vi "QCA - DUT Receive.vi"(0 "CART TCP Connection In":refnum<k5>, 1 "Rx_Test Parameters":T1 {"OFDM Data Rate (Mbps)" items=["6", "9", "12", "18", "24", "36", "48", "54"]; "DSSS Data Rate (Mbps)" items=["1", "2", "5.5 CCK", "5.5 PBCC", "11 CCK", "11 PBCC", "22", "33"]; "80211n PLCP Frame Format" items=["Mixed Format", "Greenfield Format"]}, 11 "error in (no error)":errorcluster) -> (4 "CART TCP Connection Out":refnum<k5>, 6 "Messages Logged":string[](array[string]), 14 "Command Sent":string, 15 "error out":errorcluster)   [LabVIEW 2011]
uses:
  TV/RW/Includes/WLAN - TV - RW - INC - RxTestParameters.ctl
  Controls/Data Rates.ctl
panel:
  in  "OFDM Data Rate (Mbps)":i32(ring) items=["6", "9", "12", "18", "24", "36", "48", "54"]
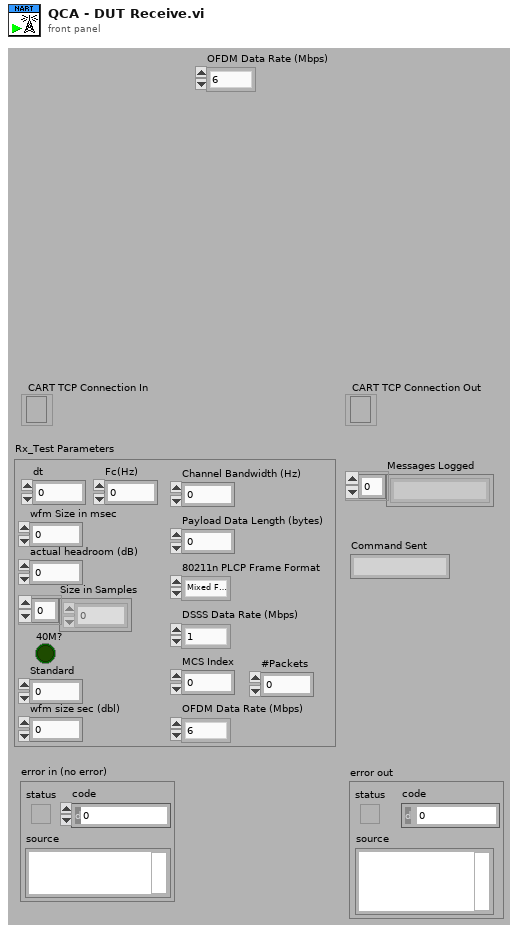
[diagram p1: front panel]
types:
  T1 = typedef "WLAN - TV - RW - INC - RxTestParameters.ctl" = cluster{"wfm Size in msec":i32, "actual headroom (dB)":dbl, "Size in Samples":i32[], "40M?":bool, "Standard ":i32, "wfm size sec (dbl)":dbl, "dt":dbl, "Channel Bandwidth (Hz)":dbl, "Payload Data Length (bytes)":i32, "80211n PLCP Frame Format":i32, "DSSS Data Rate (Mbps)":i32, "OFDM Data Rate (Mbps)":i32, "MCS Index":i32, "Fc(Hz)":dbl, "#Packets":i32}
  T2 = typedef "Data Rates.ctl" = string
  T3 = cluster{"Frequency, MHz":u32, "Data Rate":T2, "Packet Count":i32, "RX Mac Address":string, "TX Mac Address":string, "BS Mac Address":string, "Packet Length":u32, "Broadcast":bool}
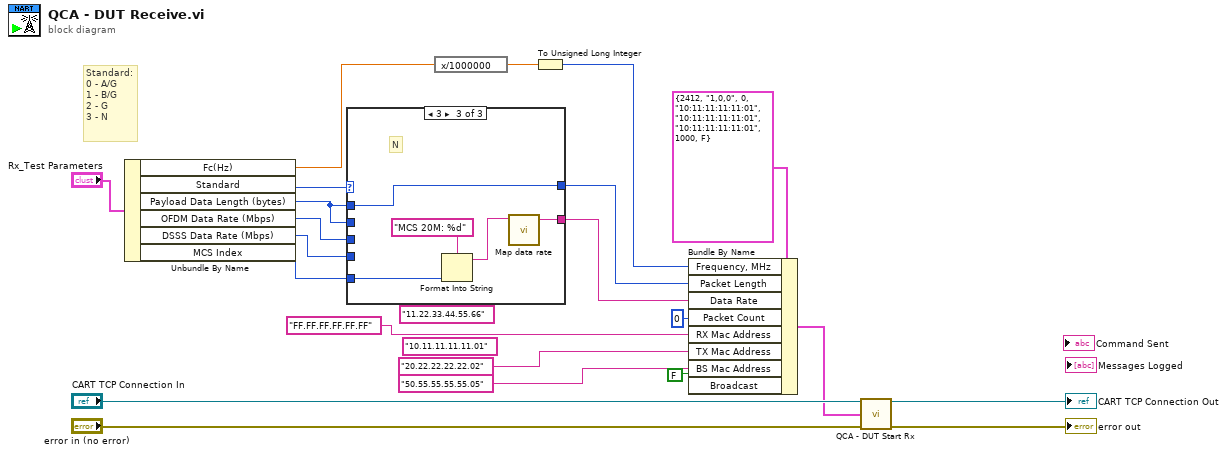
[diagram p0: block diagram]
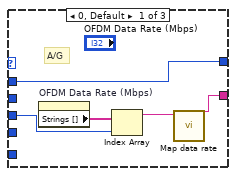
[diagram p2: hidden frame]
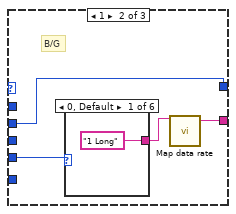
[diagram p3: hidden frame]
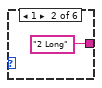
[diagram p4: hidden frame]
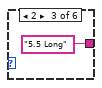
[diagram p5: hidden frame]
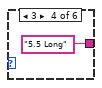
[diagram p6: hidden frame]
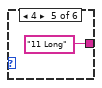
[diagram p7: hidden frame]
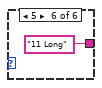
[diagram p8: hidden frame]
diagram:
  (unwired) "11.22.33.44.55.66" ("RX Mac")
  (unwired) "10.11.11.11.11.01" ("RX Mac")
  # "Standard:\n0 - A/G\n1 - B/G\n2 - G\n3 - N"
  n1 = Unbundle By Name("Rx_Test Parameters") -> ("Fc(Hz)"=w4:dbl, "Standard"=w12:i32, "Payload Data Length (bytes)"=w11:i32, "OFDM Data Rate (Mbps)"=w10:i32, "DSSS Data Rate (Mbps)"=w9:i32, "MCS Index"=w8:i32)
  n2 = case shown="3" w12 {
    tunnel: [w27 w31 w42] -> w7
    tunnel: w11 -> [w27 _ w42]
    tunnel: w11 -> [_ w31 _]
    tunnel: w10 -> [w23 _ _]
    tunnel: w9 -> [_ w30 _]
    tunnel: w8 -> [_ _ w40]
    tunnel: [w26 w29 w41] -> w6
    frame 0, Default {
      # "A/G"
      n3 = property on="OFDM Data Rate (Mbps)" class="Ring (strict)"() -> ("Strings []"=w25:string[])  [unwired: 2 in, 2 out]
      n4 = Index Array(array=w25, index=w23) -> (element=w24:string)
      n5 = call "Map data rate.vi"("Data Rate In"=w24) -> ("Data Rate Out"=w26:string)  [unwired: 10 in]
    }
    frame 1 {
      # "B/G"
      n6 = case shown="0, Default" w30 {
        tunnel: ["1 Long" ("Data Rate In") "2 Long" ("Data Rate In") "5.5 Long" ("Data Rate In") "5.5 Long" ("Data Rate In") "11 Long" ("Data Rate In") "11 Long" ("Data Rate In")] -> w28
        frame 0, Default {
        }
        frame 1 {
        }
        frame 2 {
        }
        frame 3 {
        }
        frame 4 {
        }
        frame 5 {
        }
      }
      n7 = call "Map data rate.vi"("Data Rate In"=w28) -> ("Data Rate Out"=w29:string)  [unwired: 10 in]
    }
    frame 3 {
      # "N"
      n8 = Format Into String(format string="MCS 20M: %d", w40) -> (resulting string=w38:string)  [unwired: 2 in, 1 out]
      n9 = call "Map data rate.vi"("Data Rate In"=w38) -> ("Data Rate Out"=w41:string)  [unwired: 10 in]
    }
  }
  n10 = expression code="x/1000000"(w4) -> (w17:dbl)
  n11 = To Unsigned Long Integer(number=w17) -> (unsigned 32bit integer=w16:u32)
  n12 = Bundle By Name(cluster=T3 {"Frequency, MHz"=2412, "Data Rate"="1,0,0", "Packet Count"=0, "RX Mac Address"="10:11:11:11:11:01", "TX Mac Address"="10:11:11:11:11:01", "BS Mac Address"="10:11:11:11:11:01", "Packet Length"=1000, "Broadcast"=FALSE} ("Receive Config"), "Frequency, MHz"=w16, "Packet Length"=w7, "Data Rate"=w6, "Packet Count"=0, "RX Mac Address"="FF.FF.FF.FF.FF.FF" ("RX Mac"), "TX Mac Address"="20.22.22.22.22.02" ("RX Mac"), "BS Mac Address"="50.55.55.55.55.05" ("RX Mac"), "Broadcast"=FALSE ("ART2 Data.Receive Config.Broadcast")) -> (w1:T3)
  n13 = call "QCA - DUT Start Rx.vi"("CART TCP Connection In"="CART TCP Connection In", "Receive Config"=w1, "error in (no error)"="error in (no error)") -> ("CART TCP Connection Out"=→"CART TCP Connection Out":refnum<k5>, "error out"=→"error out":errorcluster)  [unwired: 10 in, 1 out]
